vi "Post-Install Custom Action.vi"(10 "Variant":variant) -> (0 "error out":errorcluster)   [LabVIEW 2020]
uses:
  <vilib>/Utility/config.llb/Write Key (Boolean).vi
  <vilib>/Utility/config.llb/NI_LVConfig.lvlib
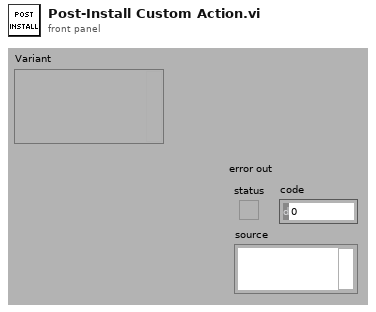
[diagram p1: front panel]
types:
  T1 = typedef "NI_LVConfig.lvlib/Config Data RefNum.ctl" = refnum<k1>
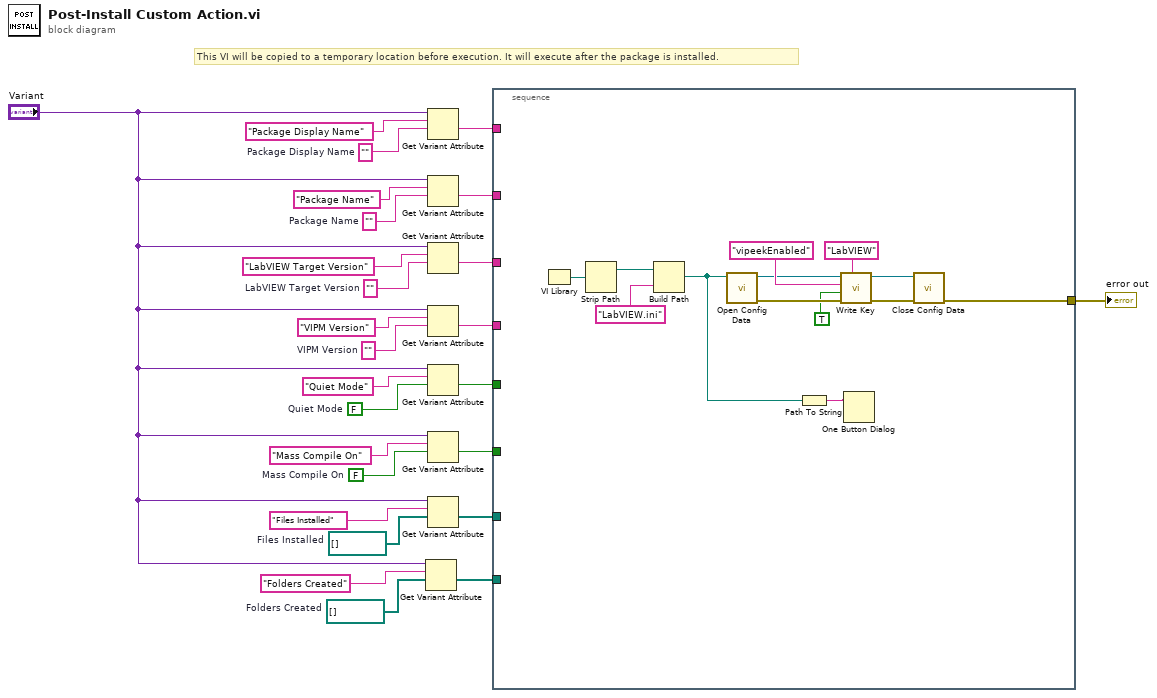
[diagram p0: block diagram]
diagram:
  w2 = path[] []  # Folders Created
  w3 = path[] []  # Files Installed
  w9 = FALSE  # Mass Compile On
  w10 = ""  # Package Display Name
  w17 = FALSE  # Quiet Mode
  w20 = ""  # VIPM Version
  w22 = ""  # LabVIEW Target Version
  w24 = ""  # Package Name
  # "This VI will be copied to a temporary location before execution. It will execute after the package is installed."
  n1 = Get Variant Attribute(Variant="Variant", name="Folders Created", default value (empty Variant)=w2) -> (value=w7:path[])  [unwired: 1 in, 3 out]
  n2 = Get Variant Attribute(Variant="Variant", name="Package Display Name", default value (empty Variant)=w10) -> (value=w16:string)  [unwired: 1 in, 3 out]
  n3 = Get Variant Attribute(Variant="Variant", name="Package Name", default value (empty Variant)=w24) -> (value=w15:string)  [unwired: 1 in, 3 out]
  n4 = Get Variant Attribute(Variant="Variant", name="LabVIEW Target Version", default value (empty Variant)=w22) -> (value=w14:string)  [unwired: 1 in, 3 out]
  n5 = Get Variant Attribute(Variant="Variant", name="VIPM Version", default value (empty Variant)=w20) -> (value=w13:string)  [unwired: 1 in, 3 out]
  n6 = Get Variant Attribute(Variant="Variant", name="Quiet Mode", default value (empty Variant)=w17) -> (value=w12:bool)  [unwired: 1 in, 3 out]
  n7 = Get Variant Attribute(Variant="Variant", name="Mass Compile On", default value (empty Variant)=w9) -> (value=w11:bool)  [unwired: 1 in, 3 out]
  n8 = Get Variant Attribute(Variant="Variant", name="Files Installed", default value (empty Variant)=w3) -> (value=w6:path[])  [unwired: 1 in, 3 out]
  n9 = stacked-sequence {
    tunnel: w16 -> [_]
    tunnel: w15 -> [_]
    tunnel: w14 -> [_]
    tunnel: w13 -> [_]
    tunnel: w12 -> [_]
    tunnel: w11 -> [_]
    tunnel: w6 -> [_]
    tunnel: w7 -> [_]
    tunnel: [w29] -> w1
    frame #0 {
      n10 = VI Library() -> (path=w39:path)
      n11 = Strip Path(path=w39) -> (stripped path=w38:path)  [unwired: 1 out]
      n12 = Build Path(base path=w38, name or relative path="LabVIEW.ini") -> (appended path=w27:path)
      n13 = call <vilib>:"Open Config Data.vi"("configuration file path"=w27) -> ("error out"=w36:errorcluster, "refnum"=w32:T1)  [unwired: 8 in, 1 out]
      n14 = Path To String(path=w27) -> (string=w28:string)
      n15 = call-poly <vilib>:"Write Key.vi"("section"="LabVIEW", "error in (no error)"=w36, "value"=TRUE, "key"="vipeekEnabled" ("section"), "refnum"=w32) -> ("error out"=w35:errorcluster, "refnum out"=w30:T1)  [unwired: 4 in, 1 out]
      n16 = One Button Dialog(message=w28) -> ()  [unwired: 1 in, 1 out]
      n17 = call <vilib>:"Close Config Data.vi"("error in (no error)"=w35, "refnum"=w30) -> ("error out"=w29:errorcluster)  [unwired: 8 in, 1 out]
    }
  }
  "error out" <- w1
